vi "Generator Randomize Infos.vi"(10 "DeviceID":T2) -> (3 "Generator_Info Array out":T1[](array[typedef]))   [LabVIEW 2018, in "IED Test Framework.lvlib" / "IED Test.lvclass"]
uses:
  IED Test.lvclass
  <vilib>/ORNL/CSEISMIC DDS/CSEISMIC DDS Base/Data Types/Controls/DeviceID.ctl
  <vilib>/ORNL/CSEISMIC DDS/CSEISMIC DDS Base/Data Types/Generator_Info.ctl
  <vilib>/ORNL/CSEISMIC DDS/CSEISMIC DDS Base/Data Types/Controls/EfficiencyCurve.ctl
  <vilib>/ORNL/CSEISMIC DDS/CSEISMIC DDS Base/CSEISMIC DDS.lvclass
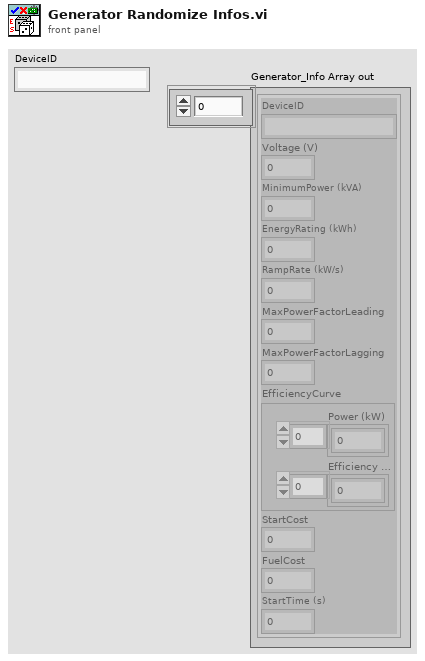
[diagram p1: front panel]
types:
  T1 = typedef "CSEISMIC DDS.lvlib/CSEISMIC DDS.lvclass/Generator_Info.ctl" = cluster{"DeviceID":T2, "Voltage (V)":dbl, "MinimumPower (kVA)":dbl, "EnergyRating (kWh)":dbl, "RampRate (kW/s)":dbl, "MaxPowerFactorLeading":dbl, "MaxPowerFactorLagging":dbl, "EfficiencyCurve":T3, "StartCost":dbl, "FuelCost":dbl, "StartTime (s)":dbl}
  T2 = typedef "CSEISMIC DDS.lvlib/CSEISMIC DDS.lvclass/DeviceID.ctl" = string
  T3 = typedef "CSEISMIC DDS.lvlib/CSEISMIC DDS.lvclass/EfficiencyCurve.ctl" = cluster{"Power (kW)":dbl[], "Efficiency (%)":dbl[]}
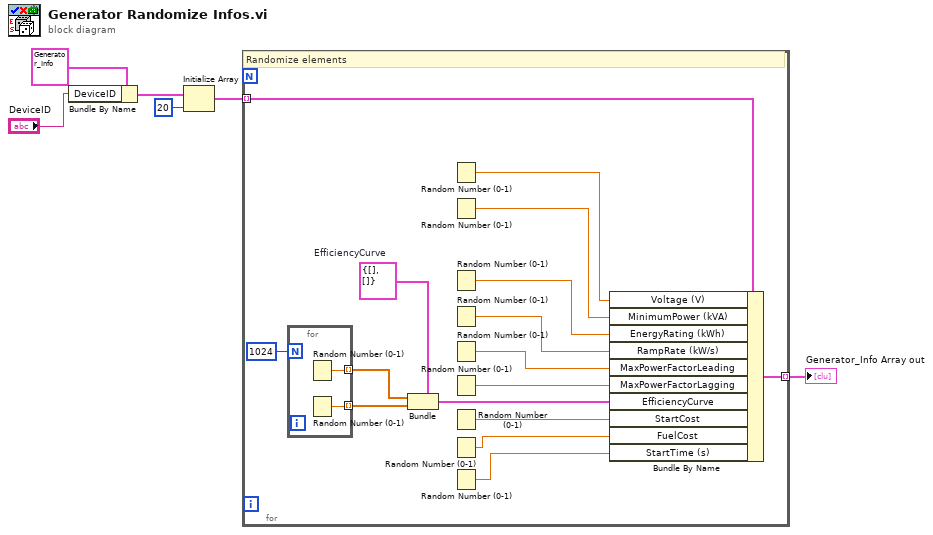
[diagram p0: block diagram]
diagram:
  n1 = Bundle By Name(cluster=T1 {"DeviceID"="", "Voltage (V)"=0.0, "MinimumPower (kVA)"=0.0, "EnergyRating (kWh)"=0.0, "RampRate (kW/s)"=0.0, "MaxPowerFactorLeading"=0.0, "MaxPowerFactorLagging"=0.0, "EfficiencyCurve"={"Power (kW)"=[], "Efficiency (%)"=[]}, "StartCost"=0.0, "FuelCost"=0.0, "StartTime (s)"=0.0} ("Generator_Info"), "DeviceID"="DeviceID") -> (w5:T1)
  n2 = Initialize Array(w5, 20 ("dimension size")) -> (w2:T1[])
  n3 = for {
    tunnel: w2 -> [w22] mode=indexing
    tunnel: [w21] -> w1 mode=indexing
    w7 = T3 {"Power (kW)"=[], "Efficiency (%)"=[]}  # EfficiencyCurve
    # "Randomize elements"
    n4 = for {
      N: 1024 -> [_]
      tunnel: [w24] -> w19 mode=indexing
      tunnel: [w23] -> w18 mode=indexing
      n5 = Random Number (0-1)() -> (number: 0 to 1=w24:dbl)
      n6 = Random Number (0-1)() -> (number: 0 to 1=w23:dbl)
    }
    n7 = Bundle(cluster=w7, "Power (kW)"=w19, "Efficiency (%)"=w18) -> (w13:T3)
    n8 = Random Number (0-1)() -> (number: 0 to 1=w17:dbl)
    n9 = Random Number (0-1)() -> (number: 0 to 1=w16:dbl)
    n10 = Random Number (0-1)() -> (number: 0 to 1=w15:dbl)
    n11 = Random Number (0-1)() -> (number: 0 to 1=w14:dbl)
    n12 = Random Number (0-1)() -> (number: 0 to 1=w12:dbl)
    n13 = Random Number (0-1)() -> (number: 0 to 1=w11:dbl)
    n14 = Random Number (0-1)() -> (number: 0 to 1=w10:dbl)
    n15 = Random Number (0-1)() -> (number: 0 to 1=w9:dbl)
    n16 = Random Number (0-1)() -> (number: 0 to 1=w8:dbl)
    n17 = Bundle By Name(cluster=w22, "Voltage (V)"=w17, "MinimumPower (kVA)"=w16, "EnergyRating (kWh)"=w15, "RampRate (kW/s)"=w14, "MaxPowerFactorLeading"=w12, "MaxPowerFactorLagging"=w11, "EfficiencyCurve"=w13, "StartCost"=w10, "FuelCost"=w9, "StartTime (s)"=w8) -> (w21:T1)
  }
  "Generator_Info Array out" <- w1
